vi "Step.vi"(7 "Path In":cluster{"Row":i32, "Col":i32}[](array[cluster]), 8 "End":cluster{"Row":i32, "Col":i32}, 10 "Grid":string[][](array[string]), 11 "Current Pos":cluster{"Row":i32, "Col":i32}) -> (3 "Paths Out":cluster{cluster{"Row":i32, "Col":i32}[]}[](array[cluster]))   [LabVIEW 2021]
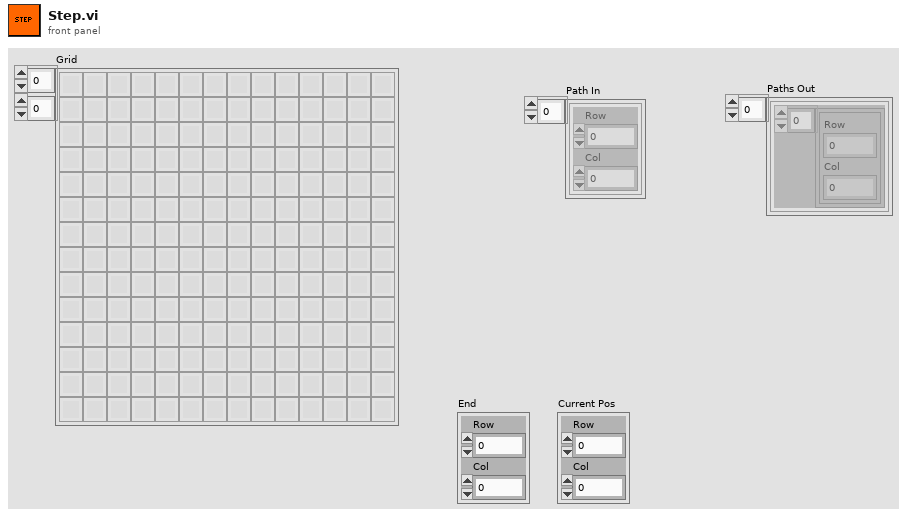
[diagram p1: front panel]
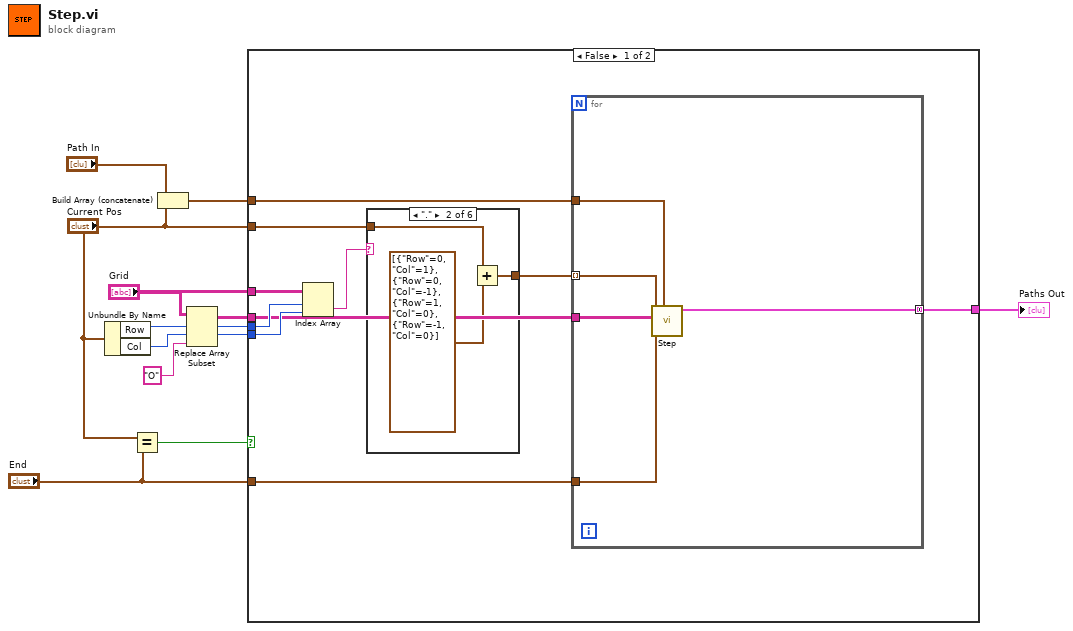
[diagram p0: block diagram]
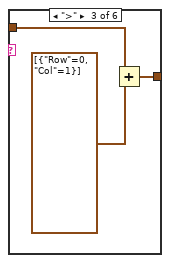
[diagram p3: hidden frame]
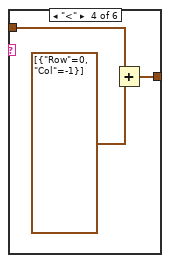
[diagram p4: hidden frame]
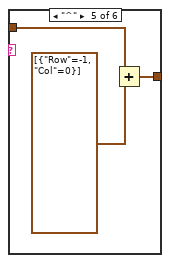
[diagram p5: hidden frame]
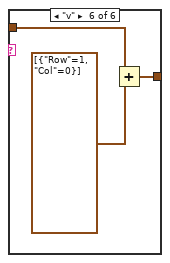
[diagram p6: hidden frame]
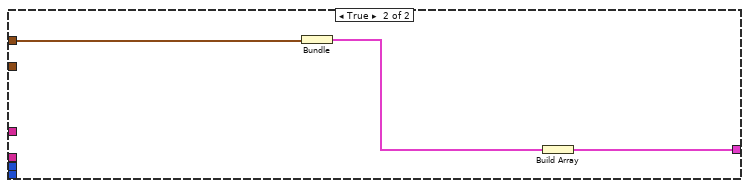
[diagram p7: hidden frame]
diagram:
  n1 = Unbundle By Name("Current Pos") -> ("Row"=w4:i32, "Col"=w3:i32)
  n2 = Equal?(x="Current Pos", y="End") -> (x = y?=w6:bool)
  n3 = Build Array (concatenate)("Path In", "Current Pos") -> (w10:cluster{"Row":i32, "Col":i32}[])
  n4 = Replace Array Subset(array="Grid", new element="O" ("new element/subarray"), index (row)=w4, index (col)=w3) -> (w7:string[][])
  n5 = case shown="False" w6 {
    tunnel: w10 -> [w21 w44]
    tunnel: [w20 w42] -> w9
    tunnel: w7 -> [w12 _]
    tunnel: "End" -> [w19 _]
    tunnel: w4 -> [w13 _]
    tunnel: w3 -> [w18 _]
    tunnel: "Current Pos" -> [w16 _]
    tunnel: "Grid" -> [w14 _]
    frame False {
      n6 = Index Array(array=w14, index (row)=w13, index (col)=w18) -> (element=w17:string)
      n7 = case shown="\".\"" w17 {
        tunnel: w16 -> [_ w24 w27 w30 w33 w36]
        tunnel: [_ w22 w25 w28 w31 w34] -> w15
        frame Default {
        }
        frame "." {
          n8 = Add(x=w24, y=cluster{"Row":i32, "Col":i32}[] [{"Row"=0, "Col"=1}, {"Row"=0, "Col"=-1}, {"Row"=1, "Col"=0}, {"Row"=-1, "Col"=0}]) -> (x+y=w22:cluster{"Row":i32, "Col":i32}[])
        }
        frame ">" {
          n9 = Add(x=w27, y=cluster{"Row":i32, "Col":i32}[] [{"Row"=0, "Col"=1}]) -> (x+y=w25:cluster{"Row":i32, "Col":i32}[])
        }
        frame "<" {
          n10 = Add(x=w30, y=cluster{"Row":i32, "Col":i32}[] [{"Row"=0, "Col"=-1}]) -> (x+y=w28:cluster{"Row":i32, "Col":i32}[])
        }
        frame "^" {
          n11 = Add(x=w33, y=cluster{"Row":i32, "Col":i32}[] [{"Row"=-1, "Col"=0}]) -> (x+y=w31:cluster{"Row":i32, "Col":i32}[])
        }
        frame "v" {
          n12 = Add(x=w36, y=cluster{"Row":i32, "Col":i32}[] [{"Row"=1, "Col"=0}]) -> (x+y=w34:cluster{"Row":i32, "Col":i32}[])
        }
      }
      n13 = for {
        tunnel: w21 -> [w39]
        tunnel: [w41] -> w20 mode=concatenating
        tunnel: w12 -> [w40]
        tunnel: w19 -> [w38]
        tunnel: w15 -> [w37] mode=indexing
        n14 = call "Step.vi"("Path In"=w39, "End"=w38, "Grid"=w40, "Current Pos"=w37) -> ("Paths Out"=w41:cluster{cluster{"Row":i32, "Col":i32}[]}[])  [unwired: 7 in]
      }
    }
    frame True {
      n15 = Bundle(w44) -> (w43:cluster{cluster{"Row":i32, "Col":i32}[]})  [unwired: 1 in]
      n16 = Build Array(w43) -> (w42:cluster{cluster{"Row":i32, "Col":i32}[]}[])
    }
  }
  "Paths Out" <- w9
